vi "motorTest.vi"() -> ()   [LabVIEW 2018]
uses:
  <instrlib>/RIGOL DS1000 Series/RIGOL DS1000 Series.lvlib
  SubVIs/Global textParse.vi
  <vilib>/measure/NI_MAPro.lvlib
  <vilib>/measure/mascope.llb/Pulse Measurements 1 chan.vi
panel:
  out "x/y 4":dbl
  out "x/y 3":dbl
  out "x/y 2":dbl
  out "x/y":dbl
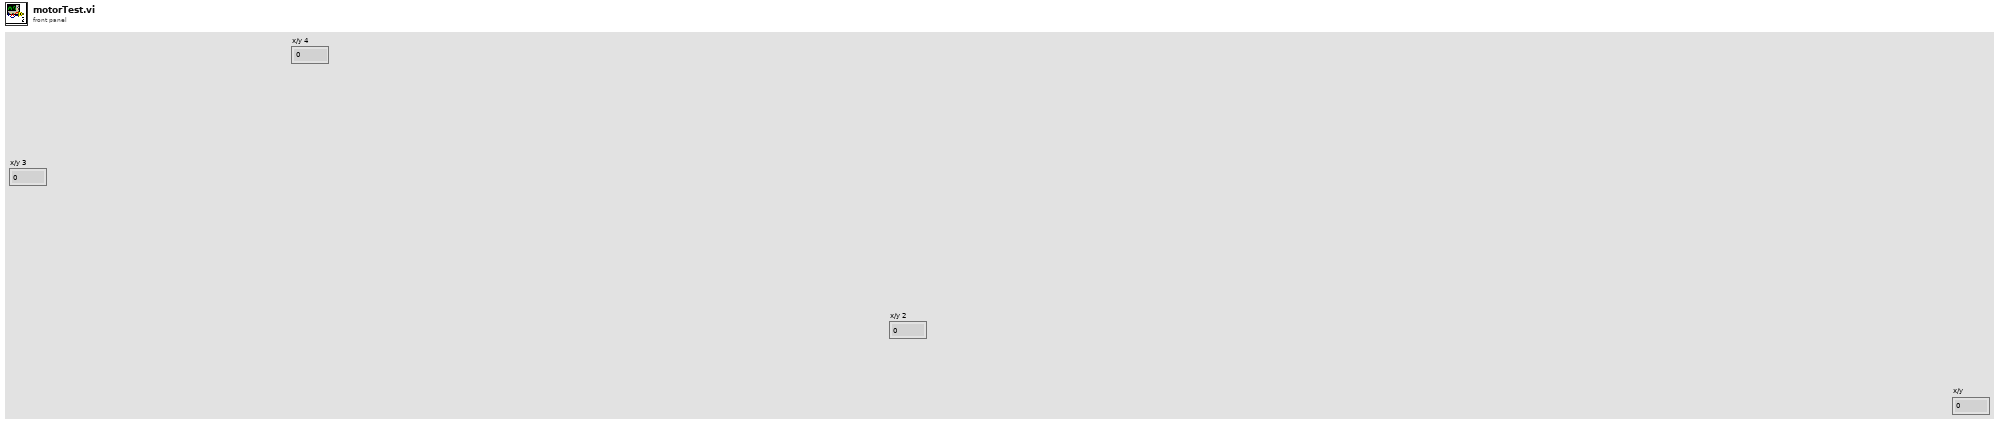
[diagram p1: front panel]
types:
  T1 = enum16{"HV", "Speed Pot", "IRcomp", "Ilimit", "Foldback", "Pass", "Fail"}
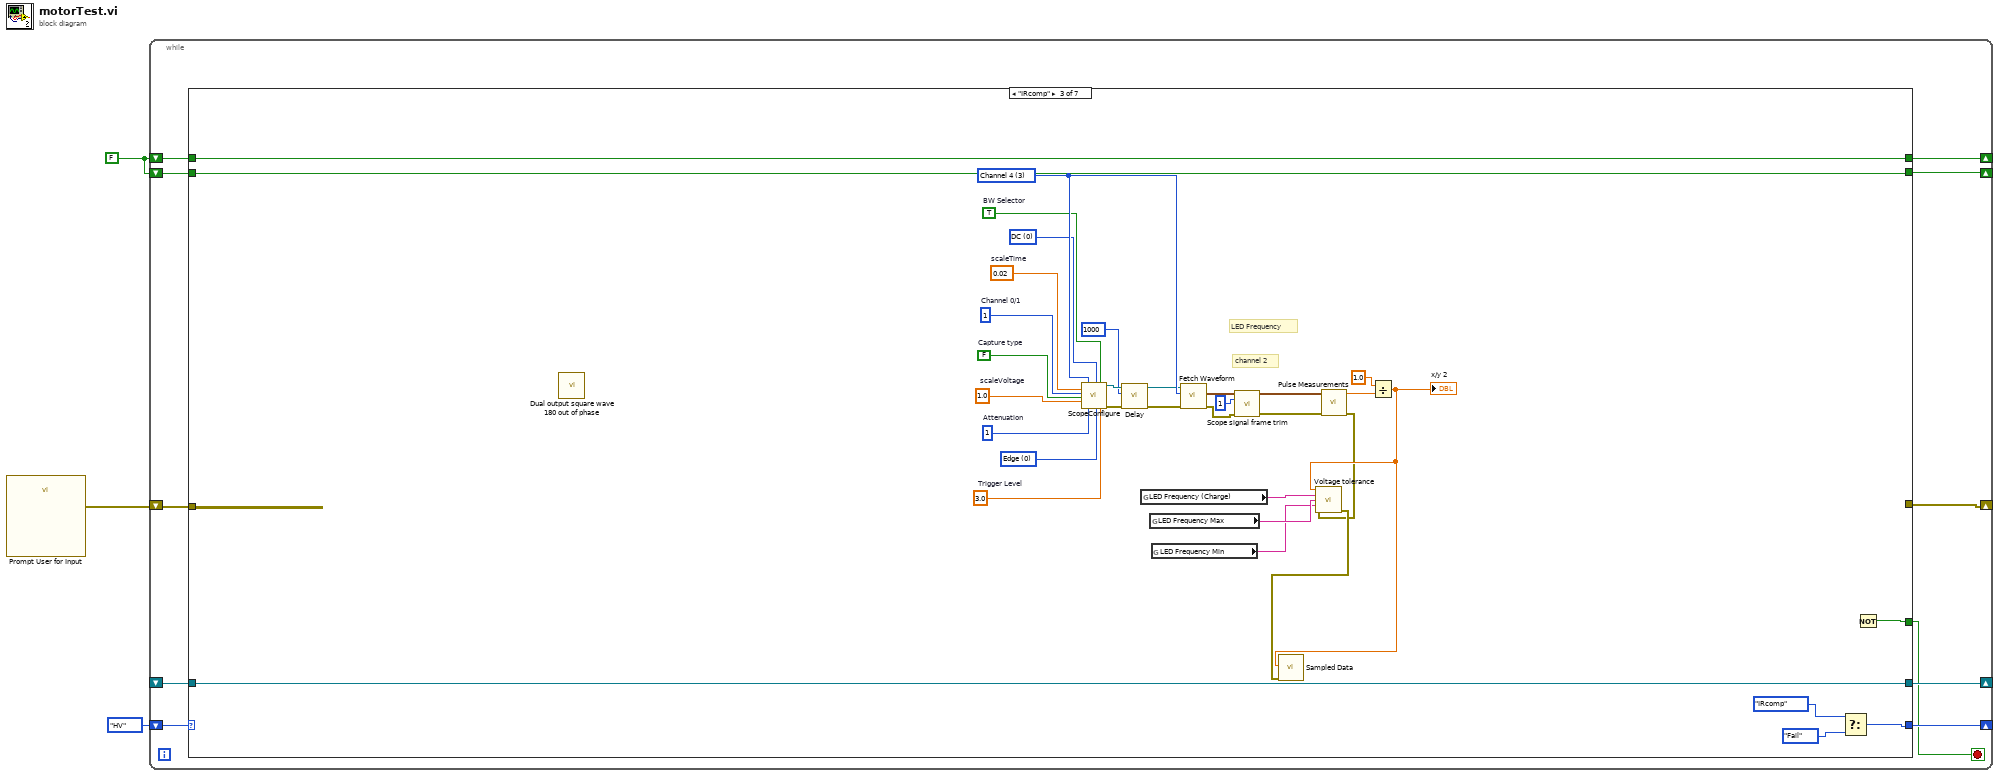
[diagram p0: block diagram]
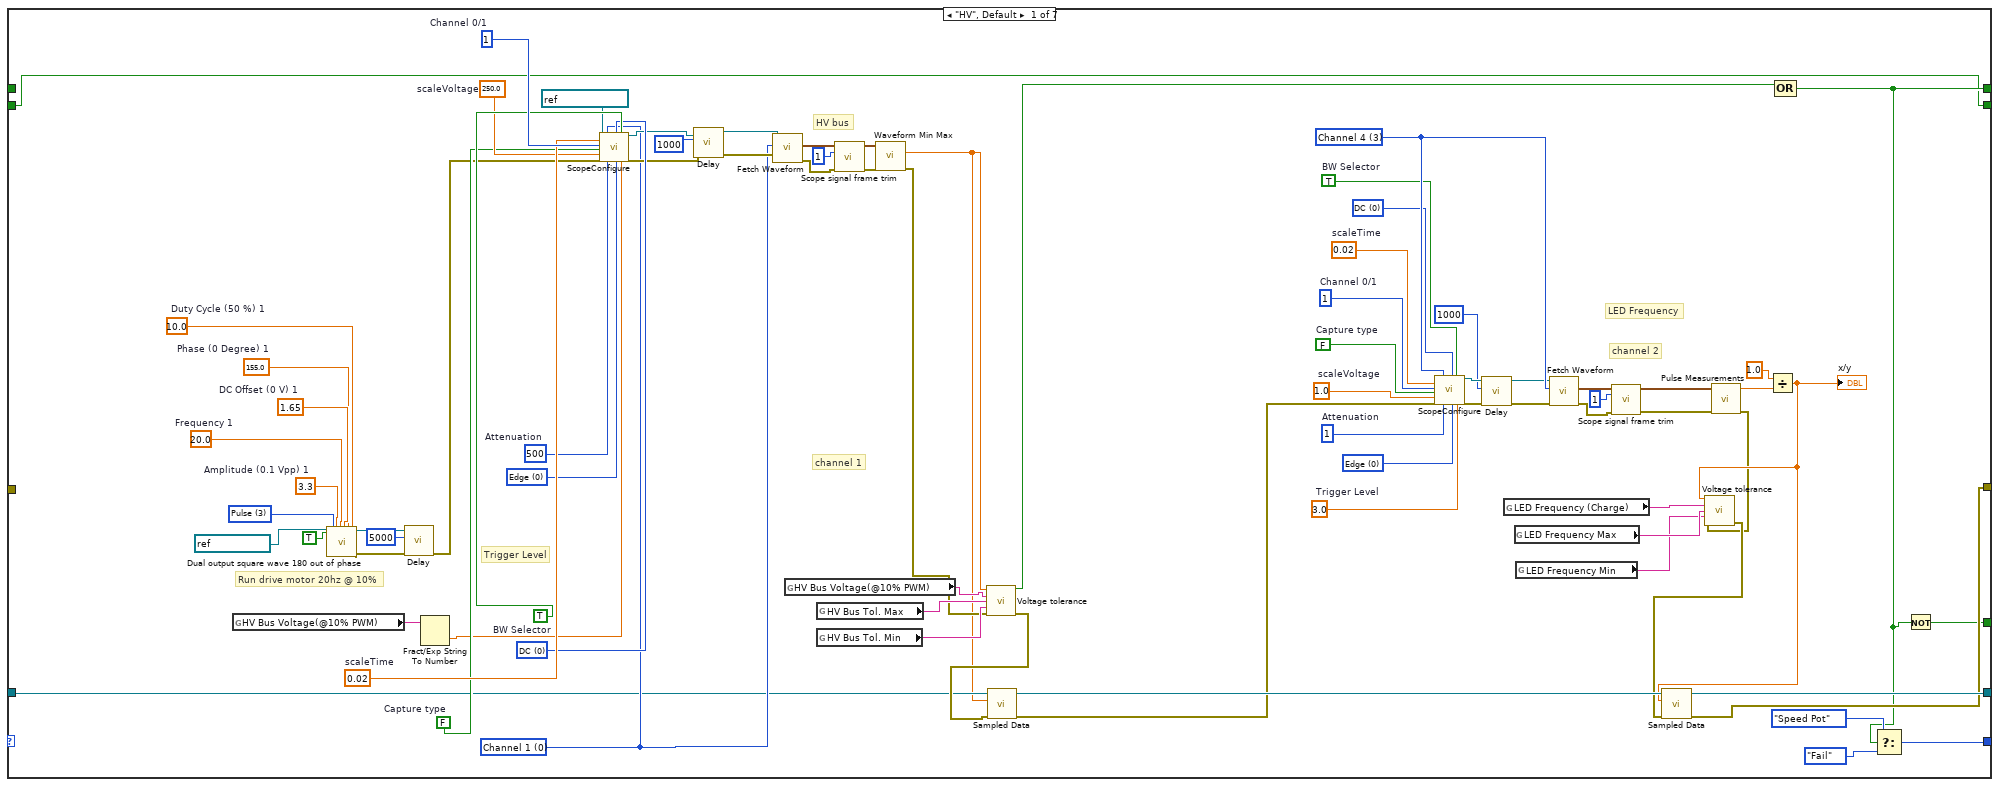
[diagram p2: hidden frame]
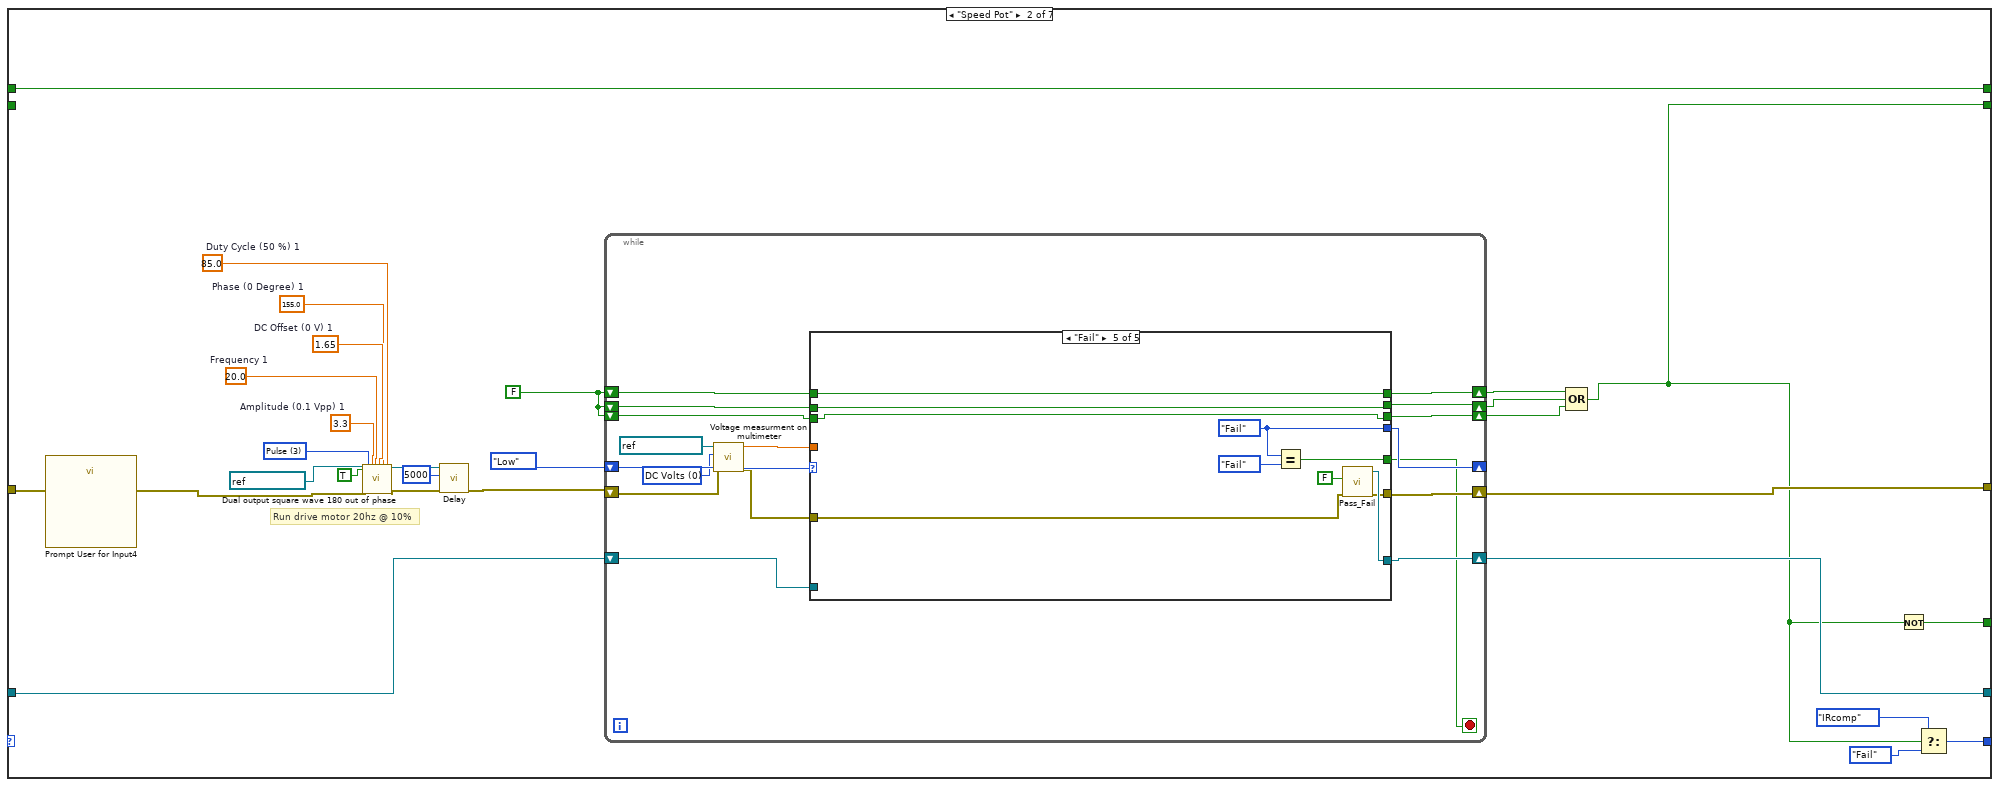
[diagram p3: hidden frame]
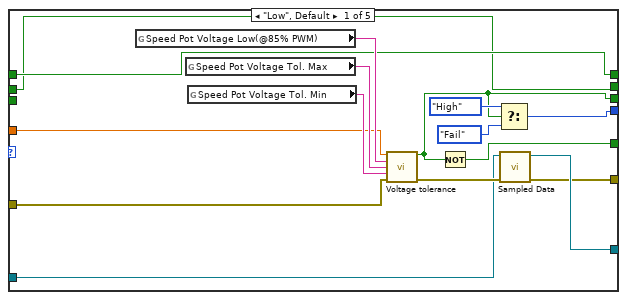
[diagram p4: hidden frame]
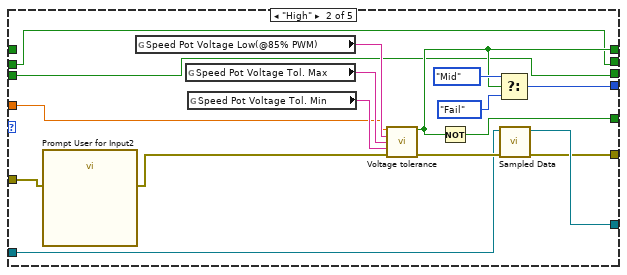
[diagram p5: hidden frame]
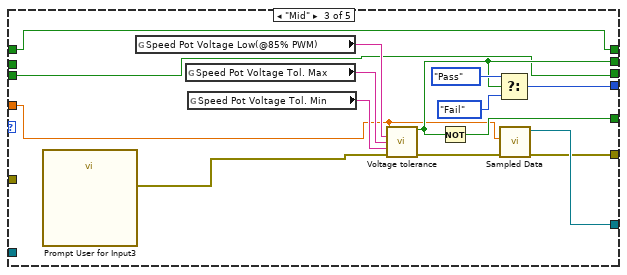
[diagram p6: hidden frame]
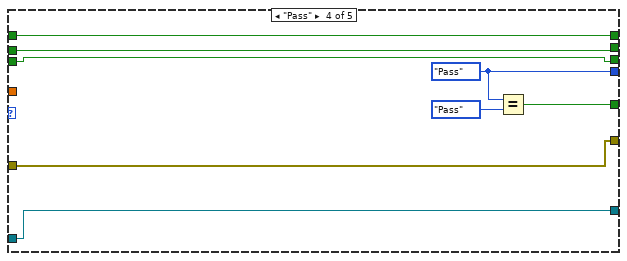
[diagram p7: hidden frame]
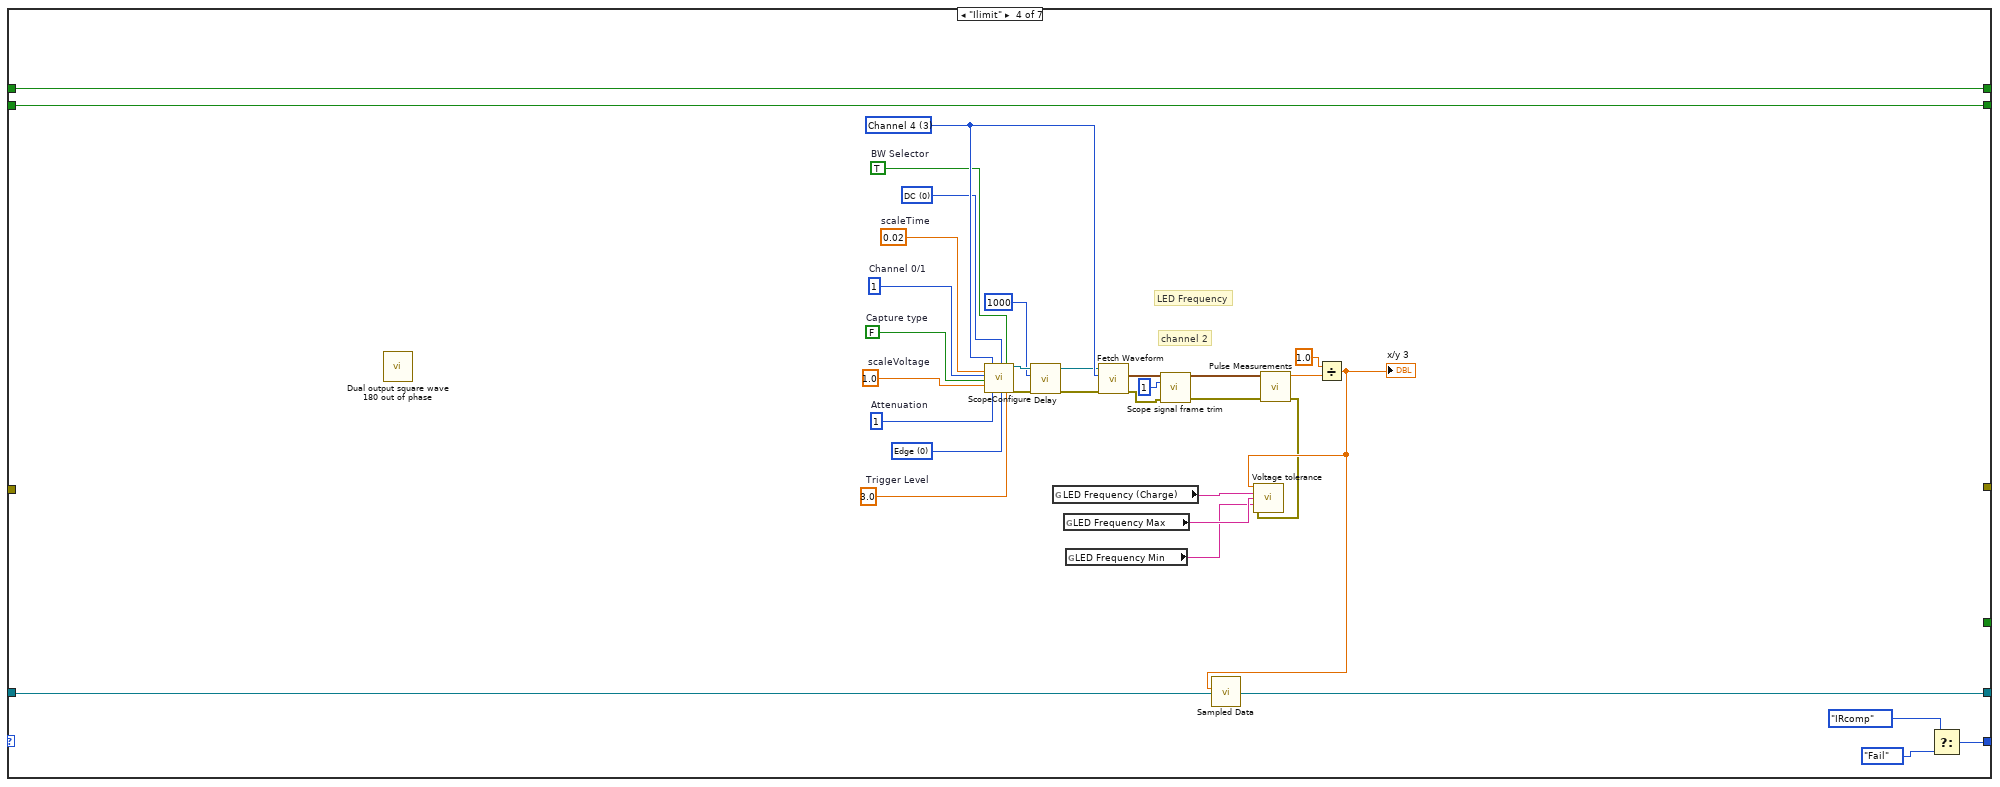
[diagram p8: hidden frame]
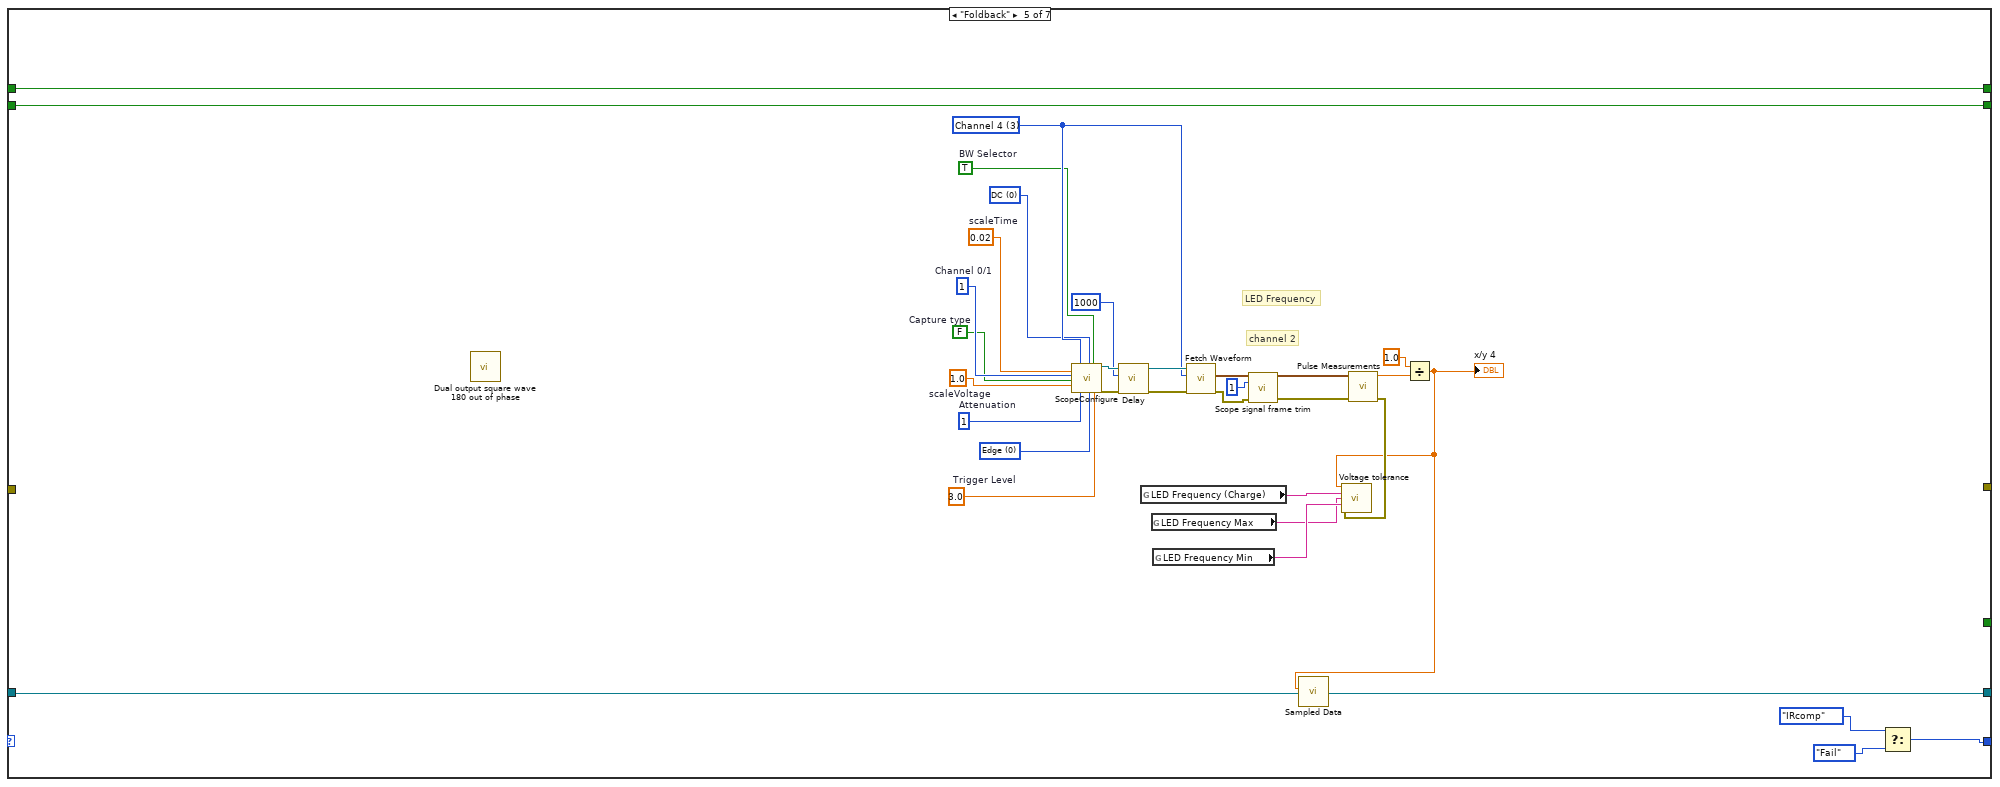
[diagram p9: hidden frame]
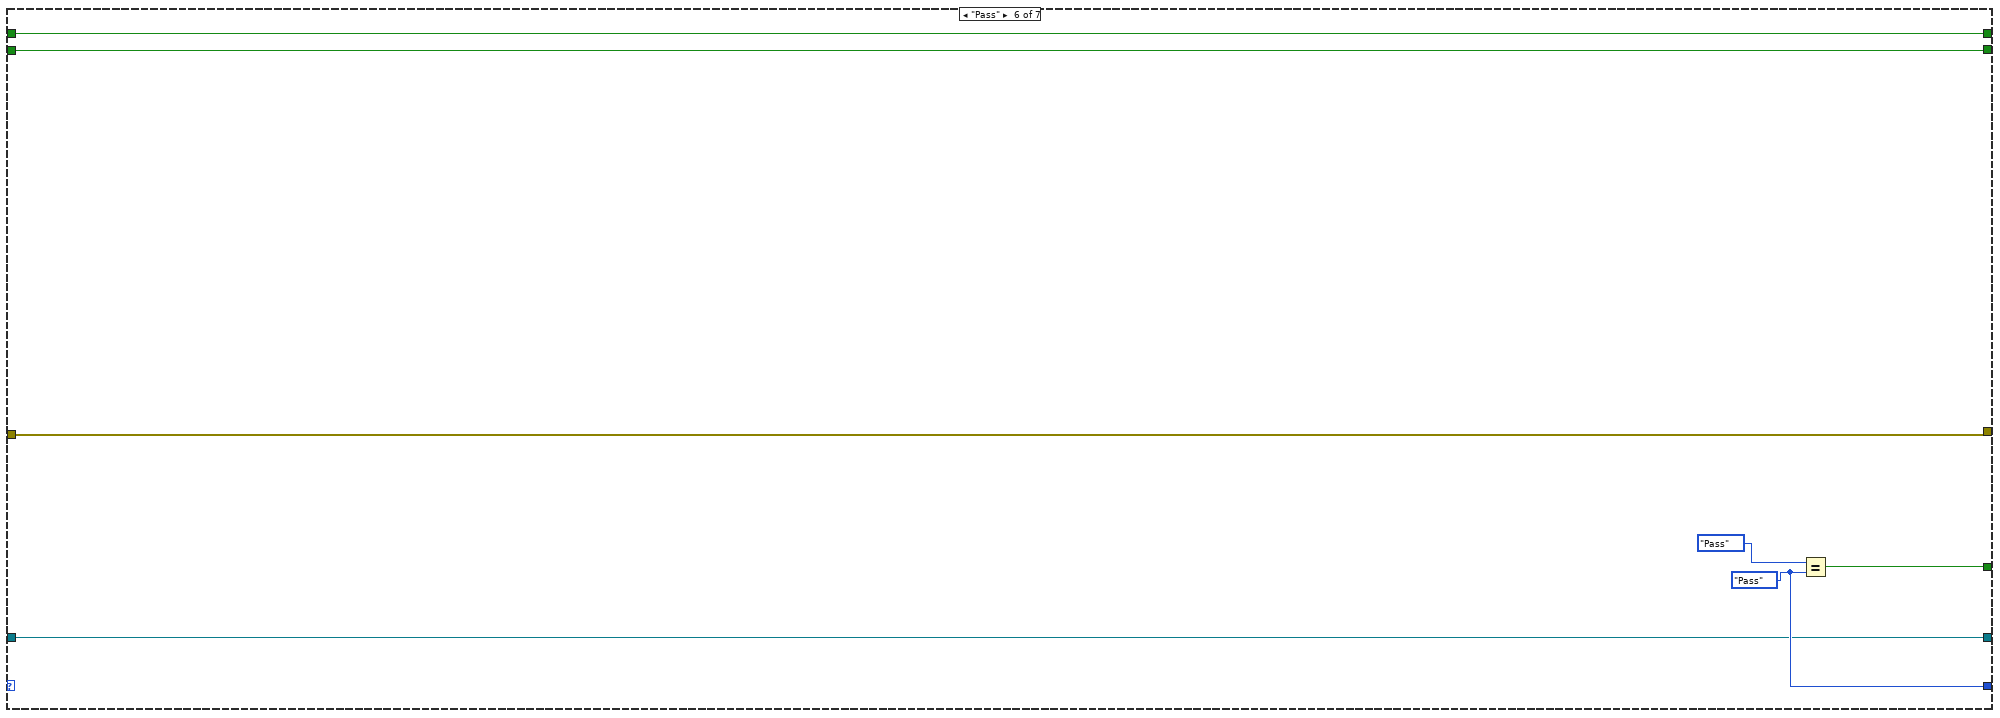
[diagram p10: hidden frame]
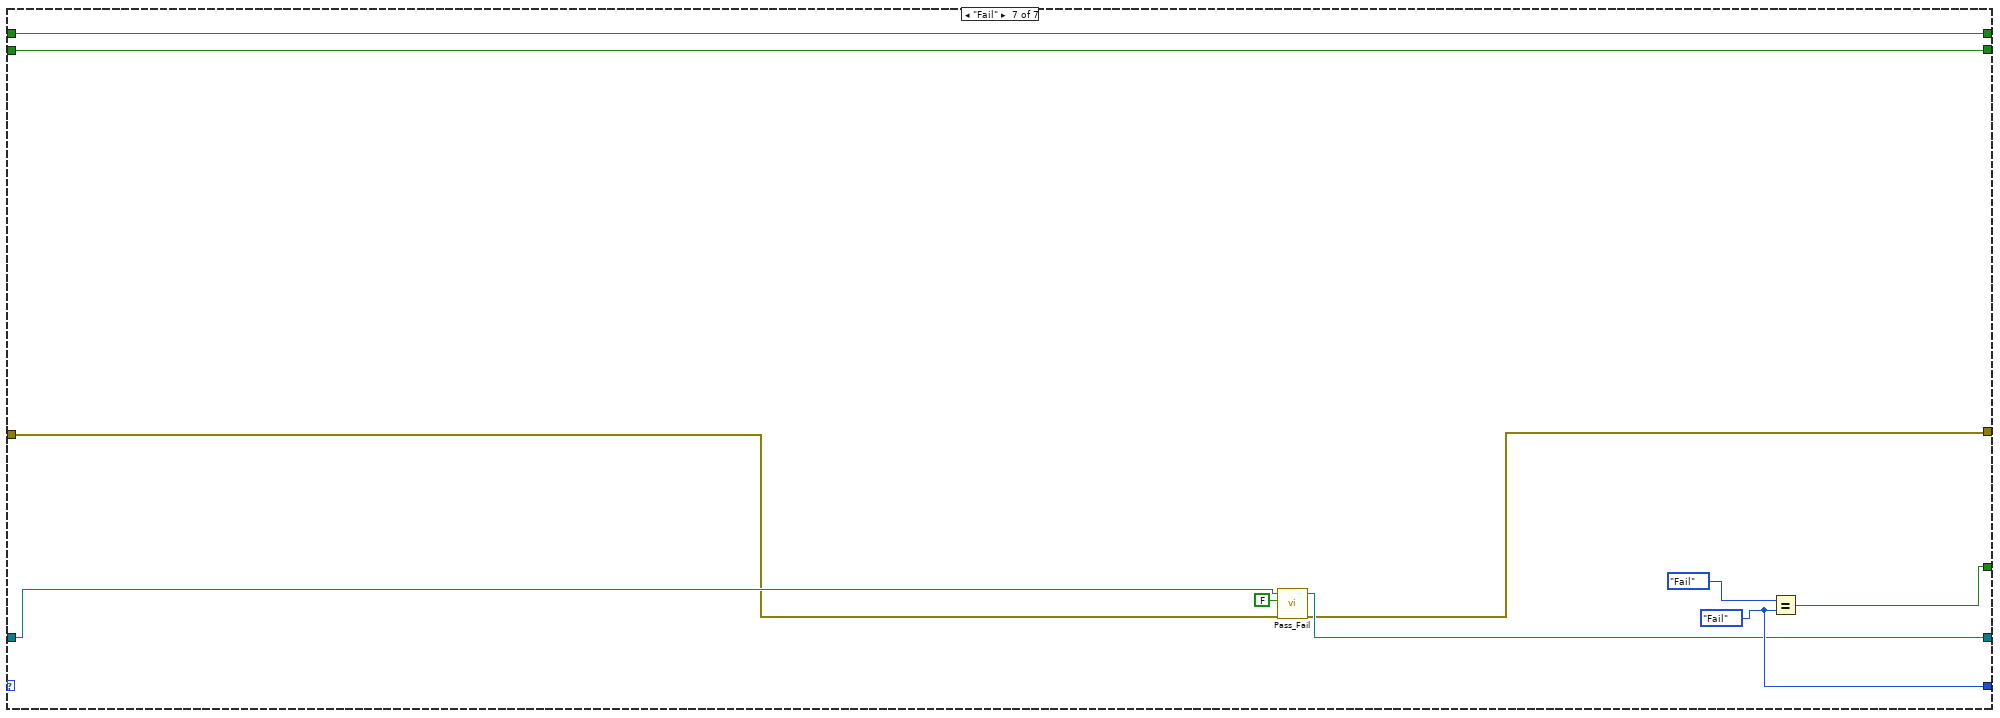
[diagram p11: hidden frame]
diagram:
  w2 = FALSE
  n1 = call "Prompt User for Input"() -> ("error out"=w1:errorcluster)  [unwired: 18 in, 1 out]
  n2 = while {
    shift-right: [w10] -> _
    shift-left: w2 -> [w12]
    shift-right: [w11] -> _
    shift-left: T1."HV" -> [w14]
    shift-right: [w8] -> _
    shift-left: _ -> [w13]
    shift-right: [w7] -> _
    shift-left: w1 -> [w9]
    shift-right: [w6] -> _
    shift-left: w2 -> [w5]
    stop <- w4 stop-if-true
    n3 = case shown="\"IRcomp\"" w14 {
      tunnel: [w51 w121 w234 w268 w301 w308 w318] -> w8
      tunnel: w13 -> [w53 w106 w234 w268 w301 w308 w315]
      tunnel: w12 -> [_ w95 w236 w273 w306 w313 w323]
      tunnel: [w57 w99 w238 w269 w302 w309 w319] -> w11
      tunnel: [w17 w95 w236 w273 w306 w313 w323] -> w10
      tunnel: [w18 w120 _ _ _ w307 w317] -> w7
      tunnel: w9 -> [_ w105 _ _ _ w307 w314]
      tunnel: [w15 w97 w235 w272 w305 w312 w322] -> w6
      tunnel: w5 -> [w15 _ w235 w272 w305 w312 w322]
      tunnel: [w16 w96 w237 _ _ w310 w320] -> w4
      frame "HV", Default {
        w33 = 1  # Channel 0/1
        w41 = FALSE  # Capture type
        w36 = u16 0 items=["Edge", "Pulse", "Video", "Pattern", "Duration"] ("Trigger Type (0: Edge)")
        w34 = 3.0  # Trigger Level
        w39 = u16 0 items=["DC", "AC", "Ground"] ("Vertical Coupling (0: DC)")
        w37 = 1  # Attenuation
        w40 = 1.0  # scaleVoltage
        w35 = 0.02  # scaleTime
        w38 = TRUE  # BW Selector
        w46 = u16 3 items=["Channel 1", "Channel 2", "Channel 3", "Channel 4"] ("Channel (0: Channel 1)")
        w82 = 1  # Channel 0/1
        w75 = FALSE  # Capture type
        w80 = u16 0 items=["Edge", "Pulse", "Video", "Pattern", "Duration"] ("Trigger Type (0: Edge)")
        w77 = u16 0 items=["DC", "AC", "Ground"] ("Vertical Coupling (0: DC)")
        w79 = 500  # Attenuation
        w76 = 250.0  # scaleVoltage
        w81 = 0.02  # scaleTime
        w78 = TRUE  # BW Selector
        w65 = u16 0 items=["Channel 1", "Channel 2", "Channel 3", "Channel 4"] ("Channel (0: Channel 1)")
        w87 = 10.0  # Duty Cycle (50 %) 1
        w88 = 155.0  # Phase (0 Degree) 1
        w94 = 1.65  # DC Offset (0 V) 1
        w93 = 20.0  # Frequency 1
        w92 = 3.3  # Amplitude (0.1 Vpp) 1
        w91 = 3 items=["Sinusoid", "Square", "Ramp", "Pulse", "Noise", "User", "Harmonic", "Custom", "DC", "AbsSine", "AbsSineHalf", "AmpALT", "AttALT", "GaussPulse", "NegRamp", "NPulse", "PPulse", "SineTra", "SineVer", "StairDn", "StairUD", "StairUp", "Trapezia", "BandLimited", "Butterworth", "Chebyshev1", "Chebyshev2", "Combin", "CPulse", "CWPulse", "DampedOsc", "DualTone", "Gamma", "GateVibr", "LEMPulse", "MCNoise", "Discharge", "Pahcur", "Quake", "Radar", "Ripple", "RoundHalf", "RoundPM", "StepResp", "SwingOsc", "TV", "Voice", "AM", "FM", "PM", "PWM", "PFM", "Cardiac", "EOG", "EEG", "EMG", "Pulseilogram", "ResSpeed", "LFPulse", "Tens1", "Tens2", "Tens3", "Lgnition", "ISO16750-2 SP", "ISO16750-2 VR", "ISO7637-2 TP1", "ISO7637-2 TP2A", "ISO7637-2 TP2B", "ISO7637-2 TP3A", "ISO7637-2 TP3B", "ISO7637-2 TP4", "ISO7637-2 TP5A", "ISO7637-2 TP5B", "SCR", "Surge", "Airy", "Besselj", "Bessely", "Cauchy", "Cubic", "Dirichlet", "Erf", "Erfc", "Erfclnv", "Erflnv", "ExpFall", "ExpRise", "Gauss", "HaverSine", "Laguerre", "Laplace", "Legend", "Log", "LogNormal", "Lorentz", "Maxwell", "Rayleigh", "Versiera", "Weibull", "ARB_X2", "CosH", "CosInt", "Cot", "CotHCon", "CotHPro", "CscCon", "CscPro", "CscHCon", "CscHPro", "RecipCon", "RecipPro", "SecCon", "SecPro", "SecH", "Sinc", "SinH", "SinInt", "Sqrt", "Tan", "TanH", "ACos", "ACosH", "ACotCon", "ACotPro", "ACotHCon", "ACotHPro", "ACscCon", "ACscPro", "ACscHCon", "ACscHPro", "ASecCon", "ASsePro", "ASecH", "ASin", "ASinH", "ATan", "ATanH", "Barlett", "BarthannWin", "Blackman", "BlackmanH", "BlackmanWin", "Boxcar", "ChebWin", "FlattopWin", "Hamming", "Hanning", "Kaiser", "NuttallWin", "ParzenWin", "TaylorWin", "Triang", "TukeyWin"] ("Waveform Shape (0: Sinusoid) 1")
        # "LED Frequency"
        # "channel 2"
        # "Run drive motor 20hz @ 10%"
        # "HV bus"
        # "Trigger Level"
        # "channel 1"
        n4 = global read "Global textParse.vi" "HV Bus Voltage(@10% PWM)"() -> (w55:string)
        n5 = call "Dual output square wave 180 out of phase.vi"("VISA resource name"=refnum<visa-resource-name> "Generator", "Enable Output 1"=TRUE, "Waveform Shape (0: Sinusoid) 1"=w91, "Amplitude (0.1 Vpp) 1"=w92, "Frequency 1"=w93, "DC Offset (0 V) 1"=w94, "Phase (0 Degree) 1"=w88, "Duty Cycle (50 %) 1"=w87) -> ("VISA resource name out"=w86:refnum<visa-resource-name>, "error out"=w85:errorcluster)  [unwired: 18 in]
        n6 = call <instrlib>:"Delay.vi"("error in (no error)"=w85, "Delay (ms)"=u32 5000, "VISA resource name"=w86) -> ("error out"=w72:errorcluster)  [unwired: 7 in, 1 out]
        n7 = Fract/Exp String To Number(string=w55) -> (number=w54:dbl)  [unwired: 3 in, 1 out]
        n8 = call "ScopeConfigure.vi"("VISA resource name"=refnum<visa-resource-name> "DemoScope", "scaleTime"=w81, "Channel 0/1"=w82, "Single Capture"=w75, "scaleVoltage"=w76, "error in (no error)"=w72, "Channel (0: Channel 1)"=w65, "Attenuation"=w79, "Vertical Coupling (0: DC)"=w77, "Trigger Type (0: Edge)"=w80, "BW Selector"=w78, "Trigger Level"=w54) -> ("VISA resource name out"=w73:refnum<visa-resource-name>, "error out"=w74:errorcluster)  [unwired: 6 in]
        n9 = call <instrlib>:"Delay.vi"("error in (no error)"=w74, "Delay (ms)"=u32 1000, "VISA resource name"=w73) -> ("error out"=w66:errorcluster, "VISA resource name out"=w67:refnum<visa-resource-name>)  [unwired: 7 in]
        n10 = call <instrlib>:"Fetch Waveform.vi"("error in (no error)"=w66, "Channel (0: Channel 1)"=w65, "VISA resource name"=w67) -> ("error out"=w20:errorcluster, "Waveform Data"=w68:waveform(dbl))  [unwired: 6 in, 1 out]
        n11 = global read "Global textParse.vi" "HV Bus Voltage(@10% PWM)"() -> (w63:string)
        n12 = global read "Global textParse.vi" "HV Bus Tol. Max"() -> (w62:string)
        n13 = global read "Global textParse.vi" "HV Bus Tol. Min"() -> (w61:string)
        n14 = call "Scope signal frame trim.vi"("Waveform Data"=w68, "Frame delete"=1, "error in (no error)"=w20) -> ("waveform out"=w69:waveform(dbl), "error out"=w19:errorcluster)  [unwired: 11 in]
        n15 = call <vilib>:"Waveform Min Max.vi"("error in (no error)"=w19, "waveform in"=w69) -> ("error out"=w60:errorcluster, "Y max"=w50:dbl)  [unwired: 4 in, 4 out]
        n16 = call "Voltage tolerance.vi"("Data Sample"=w50, "Spec Output"=w63, "Upper"=w62, "Lower"=w61, "error in (no error)"=w60) -> ("Boolean"=w59:bool, "error out"=w64:errorcluster)  [unwired: 9 in]
        n17 = call "Sampled Data.vi"("Error In"=w64, "Data Sample"=w50, "refnum in"=w53) -> ("error out"=w21:errorcluster, "refnum out"=w52:refnum<file>)  [unwired: 7 in]
        n18 = call "ScopeConfigure.vi"("scaleTime"=w35, "Channel 0/1"=w33, "Single Capture"=w41, "scaleVoltage"=w40, "error in (no error)"=w21, "Channel (0: Channel 1)"=w46, "Attenuation"=w37, "Vertical Coupling (0: DC)"=w39, "Trigger Type (0: Edge)"=w36, "BW Selector"=w38, "Trigger Level"=w34) -> ("VISA resource name out"=w43:refnum<visa-resource-name>, "error out"=w42:errorcluster)  [unwired: 7 in]
        n19 = call <instrlib>:"Delay.vi"("error in (no error)"=w42, "Delay (ms)"=u32 1000, "VISA resource name"=w43) -> ("error out"=w45:errorcluster, "VISA resource name out"=w44:refnum<visa-resource-name>)  [unwired: 7 in]
        n20 = global read "Global textParse.vi" "LED Frequency (Charge)"() -> (w49:string)
        n21 = global read "Global textParse.vi" "LED Frequency Max"() -> (w48:string)
        n22 = global read "Global textParse.vi" "LED Frequency Min"() -> (w47:string)
        n23 = call <instrlib>:"Fetch Waveform.vi"("error in (no error)"=w45, "Channel (0: Channel 1)"=w46, "VISA resource name"=w44) -> ("error out"=w26:errorcluster, "Waveform Data"=w31:waveform(dbl))  [unwired: 6 in, 1 out]
        n24 = call "Scope signal frame trim.vi"("Waveform Data"=w31, "Frame delete"=1, "error in (no error)"=w26) -> ("waveform out"=w28:waveform(dbl), "error out"=w25:errorcluster)  [unwired: 11 in]
        n25 = call-poly <vilib>:"Pulse Measurements.vi"("error in (no error)"=w25, "signal in"=w28) -> ("error out"=w22:errorcluster, "period"=w30:dbl)  [unwired: 5 in, 3 out]
        n26 = Divide(x=1.0, y=w30) -> (x/y=w24:dbl)
        "x/y" <- w24
        n27 = call "Voltage tolerance.vi"("Data Sample"=w24, "Spec Output"=w49, "Upper"=w48, "Lower"=w47, "error in (no error)"=w22) -> ("error out"=w23:errorcluster)  [unwired: 9 in, 1 out]
        n28 = call "Sampled Data.vi"("Error In"=w23, "Data Sample"=w24, "refnum in"=w52) -> ("error out"=w18:errorcluster, "refnum out"=w51:refnum<file>)  [unwired: 7 in]
        n29 = Compound Arithmetic op=OR(w59) -> (w17:bool)  [unwired: 1 in]
        n30 = Select(t=T1."Speed Pot", s=w17, f=T1."Fail") -> (s? t:f=w57:T1)
        n31 = Not(x=w17) -> (.not. x?=w16:bool)
      }
      frame "Speed Pot" {
        w111 = 85.0  # Duty Cycle (50 %) 1
        w112 = 155.0  # Phase (0 Degree) 1
        w118 = 1.65  # DC Offset (0 V) 1
        w117 = 20.0  # Frequency 1
        w116 = 3.3  # Amplitude (0.1 Vpp) 1
        w115 = 3 items=["Sinusoid", "Square", "Ramp", "Pulse", "Noise", "User", "Harmonic", "Custom", "DC", "AbsSine", "AbsSineHalf", "AmpALT", "AttALT", "GaussPulse", "NegRamp", "NPulse", "PPulse", "SineTra", "SineVer", "StairDn", "StairUD", "StairUp", "Trapezia", "BandLimited", "Butterworth", "Chebyshev1", "Chebyshev2", "Combin", "CPulse", "CWPulse", "DampedOsc", "DualTone", "Gamma", "GateVibr", "LEMPulse", "MCNoise", "Discharge", "Pahcur", "Quake", "Radar", "Ripple", "RoundHalf", "RoundPM", "StepResp", "SwingOsc", "TV", "Voice", "AM", "FM", "PM", "PWM", "PFM", "Cardiac", "EOG", "EEG", "EMG", "Pulseilogram", "ResSpeed", "LFPulse", "Tens1", "Tens2", "Tens3", "Lgnition", "ISO16750-2 SP", "ISO16750-2 VR", "ISO7637-2 TP1", "ISO7637-2 TP2A", "ISO7637-2 TP2B", "ISO7637-2 TP3A", "ISO7637-2 TP3B", "ISO7637-2 TP4", "ISO7637-2 TP5A", "ISO7637-2 TP5B", "SCR", "Surge", "Airy", "Besselj", "Bessely", "Cauchy", "Cubic", "Dirichlet", "Erf", "Erfc", "Erfclnv", "Erflnv", "ExpFall", "ExpRise", "Gauss", "HaverSine", "Laguerre", "Laplace", "Legend", "Log", "LogNormal", "Lorentz", "Maxwell", "Rayleigh", "Versiera", "Weibull", "ARB_X2", "CosH", "CosInt", "Cot", "CotHCon", "CotHPro", "CscCon", "CscPro", "CscHCon", "CscHPro", "RecipCon", "RecipPro", "SecCon", "SecPro", "SecH", "Sinc", "SinH", "SinInt", "Sqrt", "Tan", "TanH", "ACos", "ACosH", "ACotCon", "ACotPro", "ACotHCon", "ACotHPro", "ACscCon", "ACscPro", "ACscHCon", "ACscHPro", "ASecCon", "ASsePro", "ASecH", "ASin", "ASinH", "ATan", "ATanH", "Barlett", "BarthannWin", "Blackman", "BlackmanH", "BlackmanWin", "Boxcar", "ChebWin", "FlattopWin", "Hamming", "Hanning", "Kaiser", "NuttallWin", "ParzenWin", "TaylorWin", "Triang", "TukeyWin"] ("Waveform Shape (0: Sinusoid) 1")
        w119 = FALSE ("Boolean")
        # "Run drive motor 20hz @ 10%"
        n32 = call "Prompt User for Input4"("error in (no error)"=w105) -> ("error out"=w98:errorcluster)  [unwired: 17 in, 1 out]
        n33 = call "Dual output square wave 180 out of phase.vi"("VISA resource name"=refnum<visa-resource-name> "Generator", "Enable Output 1"=TRUE, "error in (no error)"=w98, "Waveform Shape (0: Sinusoid) 1"=w115, "Amplitude (0.1 Vpp) 1"=w116, "Frequency 1"=w117, "DC Offset (0 V) 1"=w118, "Phase (0 Degree) 1"=w112, "Duty Cycle (50 %) 1"=w111) -> ("VISA resource name out"=w110:refnum<visa-resource-name>, "error out"=w109:errorcluster)  [unwired: 17 in]
        n34 = call <instrlib>:"Delay.vi"("error in (no error)"=w109, "Delay (ms)"=u32 5000, "VISA resource name"=w110) -> ("error out"=w107:errorcluster)  [unwired: 7 in, 1 out]
        n35 = while {
          shift-right: [w131] -> _
          shift-left: enum16{"Low", "High", "Mid", "Pass", "Fail"}."Low" -> [w139]
          shift-right: [w137] -> w120
          shift-left: w107 -> [w135]
          shift-right: [w138] -> w121
          shift-left: w106 -> [w136]
          shift-right: [w128] -> w102
          shift-left: w119 -> [w124]
          shift-right: [w129] -> w103
          shift-left: w119 -> [w125]
          shift-right: [w130] -> w104
          shift-left: w119 -> [w126]
          stop <- w123 stop-if-true
          w133 = u16 0 items=["DC Volts", "AC Volts", "DC Current", "AC Current", "2-Wire Resistance", "4-Wire Resistance"] ("Function (0: DC Volts) 2")
          n36 = call "Voltage measurment on multimeter.vi"("error in (no error)"=w135, "Function (0: DC Volts) 2"=w133, "VISA resource name 3"=refnum<visa-resource-name> "Multimeter" ("VISA resource name out")) -> ("error out"=w134:errorcluster, "Digital Display"=w132:dbl)  [unwired: 7 in]
          n37 = case shown="\"Fail\"" w139 {
            tunnel: [w152 w169 w181 w189 w205] -> w138
            tunnel: [w141 w157 w178 w191 w198] -> w129
            tunnel: [w146 w156 w175 w190 w197] -> w128
            tunnel: [w142 w163 w176 w192 w199] -> w130
            tunnel: [w151 w165 w180 w188 w204] -> w137
            tunnel: [w150 w168 w184 w195 w202] -> w131
            tunnel: [w145 w162 w177 w193 w200] -> w123
            tunnel: w134 -> [w144 w161 _ w188 w196]
            tunnel: w136 -> [w140 w160 _ w189 _]
            tunnel: w132 -> [w143 w159 w173 _ _]
            tunnel: w126 -> [w142 _ w176 w192 w199]
            tunnel: w125 -> [w141 w157 _ w191 w198]
            tunnel: w124 -> [_ w156 w175 w190 w197]
            frame "Low", Default {
              n38 = global read "Global textParse.vi" "Speed Pot Voltage Low(@85% PWM)"() -> (w153:string)
              n39 = global read "Global textParse.vi" "Speed Pot Voltage Tol. Max"() -> (w154:string)
              n40 = global read "Global textParse.vi" "Speed Pot Voltage Tol. Min"() -> (w155:string)
              n41 = call "Voltage tolerance.vi"("Data Sample"=w143, "Spec Output"=w153, "Upper"=w154, "Lower"=w155, "error in (no error)"=w144) -> ("Boolean"=w146:bool, "error out"=w147:errorcluster)  [unwired: 9 in]
              n42 = Not(x=w146) -> (.not. x?=w145:bool)
              n43 = Select(t=enum16{"Low", "High", "Mid", "Pass", "Fail"}."High", s=w146, f=enum16{"Low", "High", "Mid", "Pass", "Fail"}."Fail") -> (s? t:f=w150:enum16{"Low", "High", "Mid", "Pass", "Fail"})
              n44 = call "Sampled Data.vi"("Error In"=w147, "refnum in"=w140) -> ("error out"=w151:errorcluster, "refnum out"=w152:refnum<file>)  [unwired: 8 in]
            }
            frame "High" {
              n45 = call "Prompt User for Input2"("error in (no error)"=w161) -> ("error out"=w158:errorcluster)  [unwired: 17 in, 1 out]
              n46 = global read "Global textParse.vi" "Speed Pot Voltage Low(@85% PWM)"() -> (w172:string)
              n47 = global read "Global textParse.vi" "Speed Pot Voltage Tol. Max"() -> (w171:string)
              n48 = global read "Global textParse.vi" "Speed Pot Voltage Tol. Min"() -> (w170:string)
              n49 = call "Voltage tolerance.vi"("Data Sample"=w159, "Spec Output"=w172, "Upper"=w171, "Lower"=w170, "error in (no error)"=w158) -> ("Boolean"=w163:bool, "error out"=w164:errorcluster)  [unwired: 9 in]
              n50 = Not(x=w163) -> (.not. x?=w162:bool)
              n51 = Select(t=enum16{"Low", "High", "Mid", "Pass", "Fail"}."Mid", s=w163, f=enum16{"Low", "High", "Mid", "Pass", "Fail"}."Fail") -> (s? t:f=w168:enum16{"Low", "High", "Mid", "Pass", "Fail"})
              n52 = call "Sampled Data.vi"("Error In"=w164, "refnum in"=w160) -> ("error out"=w165:errorcluster, "refnum out"=w169:refnum<file>)  [unwired: 8 in]
            }
            frame "Mid" {
              n53 = call "Prompt User for Input3"() -> ("error out"=w174:errorcluster)  [unwired: 18 in, 1 out]
              n54 = global read "Global textParse.vi" "Speed Pot Voltage Low(@85% PWM)"() -> (w185:string)
              n55 = global read "Global textParse.vi" "Speed Pot Voltage Tol. Max"() -> (w186:string)
              n56 = global read "Global textParse.vi" "Speed Pot Voltage Tol. Min"() -> (w187:string)
              n57 = call "Voltage tolerance.vi"("Data Sample"=w173, "Spec Output"=w185, "Upper"=w186, "Lower"=w187, "error in (no error)"=w174) -> ("Boolean"=w178:bool, "error out"=w179:errorcluster)  [unwired: 9 in]
              n58 = Not(x=w178) -> (.not. x?=w177:bool)
              n59 = Select(t=enum16{"Low", "High", "Mid", "Pass", "Fail"}."Pass", s=w178, f=enum16{"Low", "High", "Mid", "Pass", "Fail"}."Fail") -> (s? t:f=w184:enum16{"Low", "High", "Mid", "Pass", "Fail"})
              n60 = call "Sampled Data.vi"("Error In"=w179, "Data Sample"=w173) -> ("error out"=w180:errorcluster, "refnum out"=w181:refnum<file>)  [unwired: 8 in]
            }
            frame "Pass" {
              w195 = enum16{"Low", "High", "Mid", "Pass", "Fail"}."Pass"
              n61 = Equal?(x=w195, y=enum16{"Low", "High", "Mid", "Pass", "Fail"}."Pass") -> (x = y?=w193:bool)
            }
            frame "Fail" {
              w202 = enum16{"Low", "High", "Mid", "Pass", "Fail"}."Fail"
              n62 = Equal?(x=w202, y=enum16{"Low", "High", "Mid", "Pass", "Fail"}."Fail") -> (x = y?=w200:bool)
              n63 = call "Pass_Fail.vi"("error in (no error)"=w196, "OK"=FALSE) -> ("error out"=w204:errorcluster, "Byte Stream File out"=w205:refnum<file>)  [unwired: 8 in]
            }
          }
        }
        n64 = Compound Arithmetic op=OR(w104, w103, w102) -> (w97:bool)
        n65 = Not(x=w97) -> (.not. x?=w96:bool)
        n66 = Select(t=T1."IRcomp", s=w97, f=T1."Fail") -> (s? t:f=w99:T1)
      }
      frame "IRcomp" {
        w217 = 1  # Channel 0/1
        w225 = FALSE  # Capture type
        w220 = u16 0 items=["Edge", "Pulse", "Video", "Pattern", "Duration"] ("Trigger Type (0: Edge)")
        w218 = 3.0  # Trigger Level
        w223 = u16 0 items=["DC", "AC", "Ground"] ("Vertical Coupling (0: DC)")
        w221 = 1  # Attenuation
        w224 = 1.0  # scaleVoltage
        w219 = 0.02  # scaleTime
        w222 = TRUE  # BW Selector
        w230 = u16 3 items=["Channel 1", "Channel 2", "Channel 3", "Channel 4"] ("Channel (0: Channel 1)")
        # "LED Frequency"
        # "channel 2"
        n67 = call "Dual output square wave 180 out of phase.vi"() -> ()  [unwired: 26 in, 2 out]
        n68 = call "ScopeConfigure.vi"("scaleTime"=w219, "Channel 0/1"=w217, "Single Capture"=w225, "scaleVoltage"=w224, "Channel (0: Channel 1)"=w230, "Attenuation"=w221, "Vertical Coupling (0: DC)"=w223, "Trigger Type (0: Edge)"=w220, "BW Selector"=w222, "Trigger Level"=w218) -> ("VISA resource name out"=w227:refnum<visa-resource-name>, "error out"=w226:errorcluster)  [unwired: 8 in]
        n69 = call <instrlib>:"Delay.vi"("error in (no error)"=w226, "Delay (ms)"=u32 1000, "VISA resource name"=w227) -> ("error out"=w229:errorcluster, "VISA resource name out"=w228:refnum<visa-resource-name>)  [unwired: 7 in]
        n70 = global read "Global textParse.vi" "LED Frequency (Charge)"() -> (w233:string)
        n71 = global read "Global textParse.vi" "LED Frequency Max"() -> (w232:string)
        n72 = global read "Global textParse.vi" "LED Frequency Min"() -> (w231:string)
        n73 = call <instrlib>:"Fetch Waveform.vi"("error in (no error)"=w229, "Channel (0: Channel 1)"=w230, "VISA resource name"=w228) -> ("error out"=w210:errorcluster, "Waveform Data"=w215:waveform(dbl))  [unwired: 6 in, 1 out]
        n74 = call "Scope signal frame trim.vi"("Waveform Data"=w215, "Frame delete"=1, "error in (no error)"=w210) -> ("waveform out"=w212:waveform(dbl), "error out"=w209:errorcluster)  [unwired: 11 in]
        n75 = call-poly <vilib>:"Pulse Measurements.vi"("error in (no error)"=w209, "signal in"=w212) -> ("error out"=w206:errorcluster, "period"=w214:dbl)  [unwired: 5 in, 3 out]
        n76 = Divide(x=1.0, y=w214) -> (x/y=w208:dbl)
        "x/y 2" <- w208
        n77 = call "Voltage tolerance.vi"("Data Sample"=w208, "Spec Output"=w233, "Upper"=w232, "Lower"=w231, "error in (no error)"=w206) -> ("error out"=w207:errorcluster)  [unwired: 9 in, 1 out]
        n78 = call "Sampled Data.vi"("Error In"=w207, "Data Sample"=w208) -> ()  [unwired: 8 in, 2 out]
        n79 = Select(t=T1."IRcomp", f=T1."Fail") -> (s? t:f=w238:T1)  [unwired: 1 in]
        n80 = Not() -> (.not. x?=w237:bool)  [unwired: 1 in]
      }
      frame "Ilimit" {
        w251 = 1  # Channel 0/1
        w259 = FALSE  # Capture type
        w254 = u16 0 items=["Edge", "Pulse", "Video", "Pattern", "Duration"] ("Trigger Type (0: Edge)")
        w252 = 3.0  # Trigger Level
        w257 = u16 0 items=["DC", "AC", "Ground"] ("Vertical Coupling (0: DC)")
        w255 = 1  # Attenuation
        w258 = 1.0  # scaleVoltage
        w253 = 0.02  # scaleTime
        w256 = TRUE  # BW Selector
        w264 = u16 3 items=["Channel 1", "Channel 2", "Channel 3", "Channel 4"] ("Channel (0: Channel 1)")
        # "LED Frequency"
        # "channel 2"
        n81 = call "Dual output square wave 180 out of phase.vi"() -> ()  [unwired: 26 in, 2 out]
        n82 = call "ScopeConfigure.vi"("scaleTime"=w253, "Channel 0/1"=w251, "Single Capture"=w259, "scaleVoltage"=w258, "Channel (0: Channel 1)"=w264, "Attenuation"=w255, "Vertical Coupling (0: DC)"=w257, "Trigger Type (0: Edge)"=w254, "BW Selector"=w256, "Trigger Level"=w252) -> ("VISA resource name out"=w261:refnum<visa-resource-name>, "error out"=w260:errorcluster)  [unwired: 8 in]
        n83 = call <instrlib>:"Delay.vi"("error in (no error)"=w260, "Delay (ms)"=u32 1000, "VISA resource name"=w261) -> ("error out"=w263:errorcluster, "VISA resource name out"=w262:refnum<visa-resource-name>)  [unwired: 7 in]
        n84 = global read "Global textParse.vi" "LED Frequency (Charge)"() -> (w267:string)
        n85 = global read "Global textParse.vi" "LED Frequency Max"() -> (w266:string)
        n86 = global read "Global textParse.vi" "LED Frequency Min"() -> (w265:string)
        n87 = call <instrlib>:"Fetch Waveform.vi"("error in (no error)"=w263, "Channel (0: Channel 1)"=w264, "VISA resource name"=w262) -> ("error out"=w244:errorcluster, "Waveform Data"=w249:waveform(dbl))  [unwired: 6 in, 1 out]
        n88 = call "Scope signal frame trim.vi"("Waveform Data"=w249, "Frame delete"=1, "error in (no error)"=w244) -> ("waveform out"=w246:waveform(dbl), "error out"=w243:errorcluster)  [unwired: 11 in]
        n89 = call-poly <vilib>:"Pulse Measurements.vi"("error in (no error)"=w243, "signal in"=w246) -> ("error out"=w241:errorcluster, "period"=w248:dbl)  [unwired: 5 in, 3 out]
        n90 = Divide(x=1.0, y=w248) -> (x/y=w242:dbl)
        "x/y 3" <- w242
        n91 = call "Sampled Data.vi"("Data Sample"=w242) -> ()  [unwired: 9 in, 2 out]
        n92 = call "Voltage tolerance.vi"("Data Sample"=w242, "Spec Output"=w267, "Upper"=w266, "Lower"=w265, "error in (no error)"=w241) -> ()  [unwired: 9 in, 2 out]
        n93 = Select(t=T1."IRcomp", f=T1."Fail") -> (s? t:f=w269:T1)  [unwired: 1 in]
      }
      frame "Foldback" {
        w285 = 1  # Channel 0/1
        w284 = FALSE  # Capture type
        w279 = u16 0 items=["Edge", "Pulse", "Video", "Pattern", "Duration"] ("Trigger Type (0: Edge)")
        w277 = 3.0  # Trigger Level
        w280 = u16 0 items=["DC", "AC", "Ground"] ("Vertical Coupling (0: DC)")
        w281 = 1  # Attenuation
        w283 = 1.0  # scaleVoltage
        w286 = 0.02  # scaleTime
        w278 = TRUE  # BW Selector
        w282 = u16 3 items=["Channel 1", "Channel 2", "Channel 3", "Channel 4"] ("Channel (0: Channel 1)")
        # "LED Frequency"
        # "channel 2"
        n94 = call "Dual output square wave 180 out of phase.vi"() -> ()  [unwired: 26 in, 2 out]
        n95 = call "ScopeConfigure.vi"("scaleTime"=w286, "Channel 0/1"=w285, "Single Capture"=w284, "scaleVoltage"=w283, "Channel (0: Channel 1)"=w282, "Attenuation"=w281, "Vertical Coupling (0: DC)"=w280, "Trigger Type (0: Edge)"=w279, "BW Selector"=w278, "Trigger Level"=w277) -> ("VISA resource name out"=w292:refnum<visa-resource-name>, "error out"=w293:errorcluster)  [unwired: 8 in]
        n96 = call <instrlib>:"Delay.vi"("error in (no error)"=w293, "Delay (ms)"=u32 1000, "VISA resource name"=w292) -> ("error out"=w290:errorcluster, "VISA resource name out"=w291:refnum<visa-resource-name>)  [unwired: 7 in]
        n97 = global read "Global textParse.vi" "LED Frequency (Charge)"() -> (w287:string)
        n98 = global read "Global textParse.vi" "LED Frequency Max"() -> (w288:string)
        n99 = global read "Global textParse.vi" "LED Frequency Min"() -> (w289:string)
        n100 = call <instrlib>:"Fetch Waveform.vi"("error in (no error)"=w290, "Channel (0: Channel 1)"=w282, "VISA resource name"=w291) -> ("error out"=w297:errorcluster, "Waveform Data"=w294:waveform(dbl))  [unwired: 6 in, 1 out]
        n101 = call "Scope signal frame trim.vi"("Waveform Data"=w294, "Frame delete"=1, "error in (no error)"=w297) -> ("waveform out"=w296:waveform(dbl), "error out"=w298:errorcluster)  [unwired: 11 in]
        n102 = call-poly <vilib>:"Pulse Measurements.vi"("error in (no error)"=w298, "signal in"=w296) -> ("error out"=w300:errorcluster, "period"=w295:dbl)  [unwired: 5 in, 3 out]
        n103 = Divide(x=1.0, y=w295) -> (x/y=w299:dbl)
        "x/y 4" <- w299
        n104 = call "Sampled Data.vi"("Data Sample"=w299) -> ()  [unwired: 9 in, 2 out]
        n105 = call "Voltage tolerance.vi"("Data Sample"=w299, "Spec Output"=w287, "Upper"=w288, "Lower"=w289, "error in (no error)"=w300) -> ()  [unwired: 9 in, 2 out]
        n106 = Select(t=T1."IRcomp", f=T1."Fail") -> (s? t:f=w302:T1)  [unwired: 1 in]
      }
      frame "Pass" {
        w309 = T1."Pass"
        n107 = Equal?(x=T1."Pass", y=w309) -> (x = y?=w310:bool)
      }
      frame "Fail" {
        w319 = T1."Fail"
        n108 = call "Pass_Fail.vi"("error in (no error)"=w314, "OK"=FALSE, "Byte Stream File in"=w315) -> ("error out"=w317:errorcluster, "Byte Stream File out"=w318:refnum<file>)  [unwired: 7 in]
        n109 = Equal?(x=T1."Fail", y=w319) -> (x = y?=w320:bool)
      }
    }
  }
